vi "AM Modulation Demo (Baseband-Sine) - Template.vi"() -> ()   [LabVIEW 2013]
uses:
  <vilib>/express/express analysis/Spectral/Block/exnSpectralBlock spectral measurements power poly.vi
  <vilib>/express/express analysis/Spectral/Block/exnSpectralBlock spectral measurements power DDT.vi
  <vilib>/express/express analysis/Spectral/XNode/ExpressSpectralMeasurementsBlockNode.xnode
panel:
  in  "WAV Sample Rate":dbl=44100.0 caption="dt"
  in  "Mod. Freq.":dbl=2000.0 caption="Frequency"
  in  "LPF Cut-Off":dbl=10000.0 caption="Lower Cut-Off"
  in  "AWGN (dB)":dbl(slide)=0.6 caption="Standard deviation" scale=-20.0..30.0
  out "Comparision":dynamicdata(graph)
  out "Baseband":dynamicdata(graph)
  out "AM FFT":dynamicdata(graph)
  out "AM Wave":dynamicdata(graph)
  in  "DC Offset":dbl=1.0
  in  "Carrier Amp.":dbl=1.0 caption="Amplitude"
  in  "stop":bool
  in  "Modulation Index":dbl(slide)=1.0 scale=0.0..5.0
  in  "Carrier Freq.":dbl=100000.0 caption="Frequency"
  out "After Rectifier":dynamicdata(graph)=[{"t0"=timestamp(0 s since 1904-01-01), "dt"=10.0, "Y"=array[50000 elements], "attributes"=variant("NI_ChannelName"=variant(string "Sine (Power Spectrum)"), "NI_ExpIsRelativeTime"=variant(bool TRUE), "NI_ExpStartTimeStamp"=variant(timestamp timestamp(3635665779.2842293 s since 1904-01-01)), "NI_ExpTimeStamp"=variant(timestamp timestamp(3635665779.2842293 s since 1904-01-01)), "NI_ExpXDimension"=variant(string "f"), "NI_OriginalChannelName"=variant(string "Sine"))}]
  # "Amplitude Modulation"
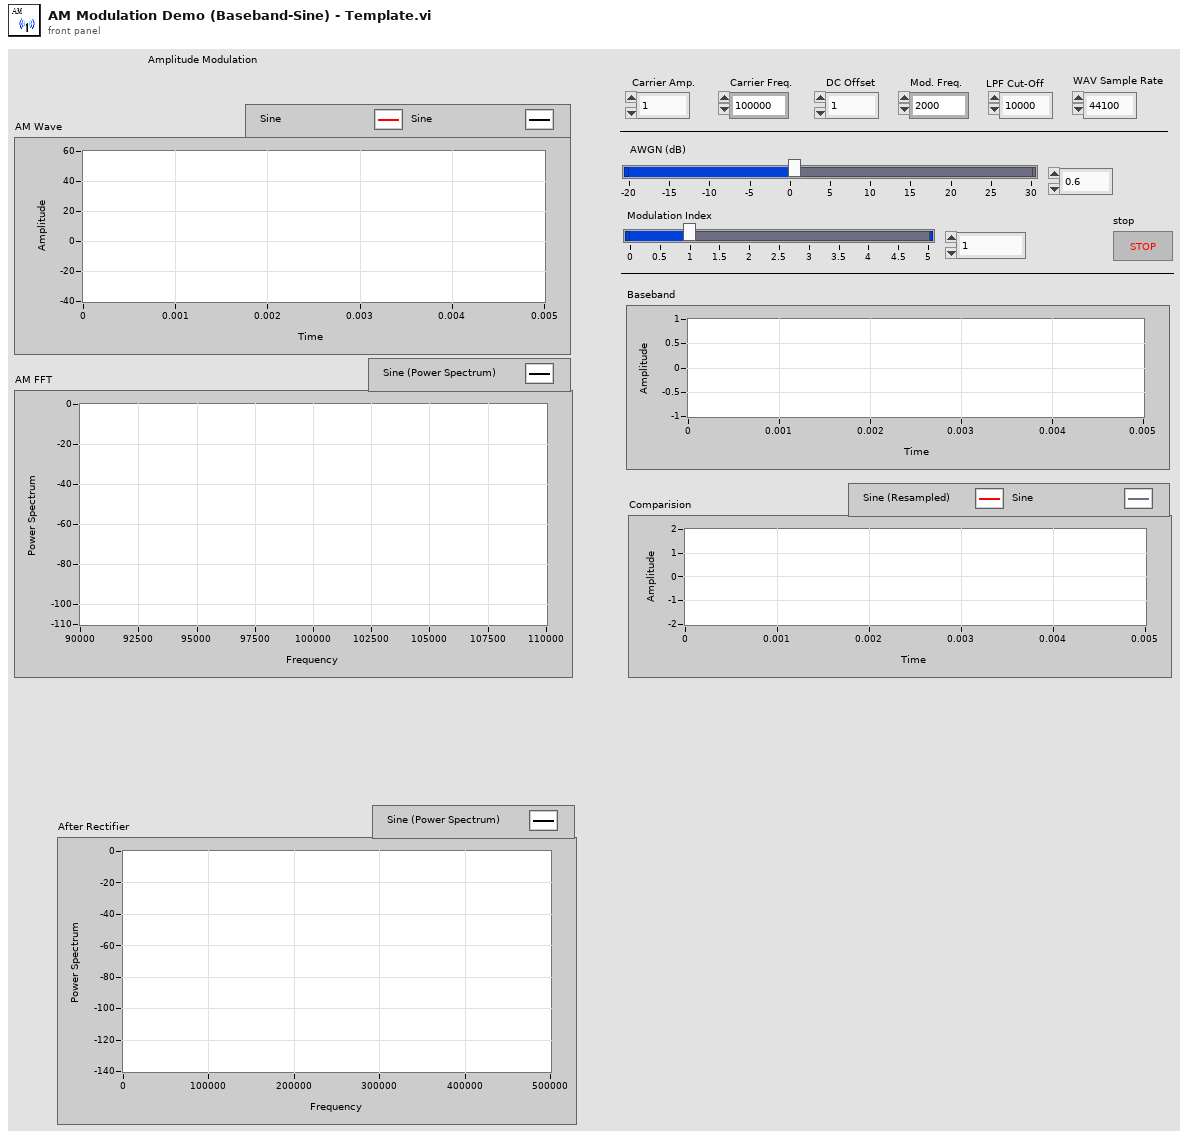
[diagram p1: front panel]
types:
  T1 = cluster{"averaging mode":u16, "weighting mode":u16, "number of averages":u32}
  T2 = cluster{"dB On (F)":bool, "unwrap phase (F)":bool, "convert to degree (F)":bool}
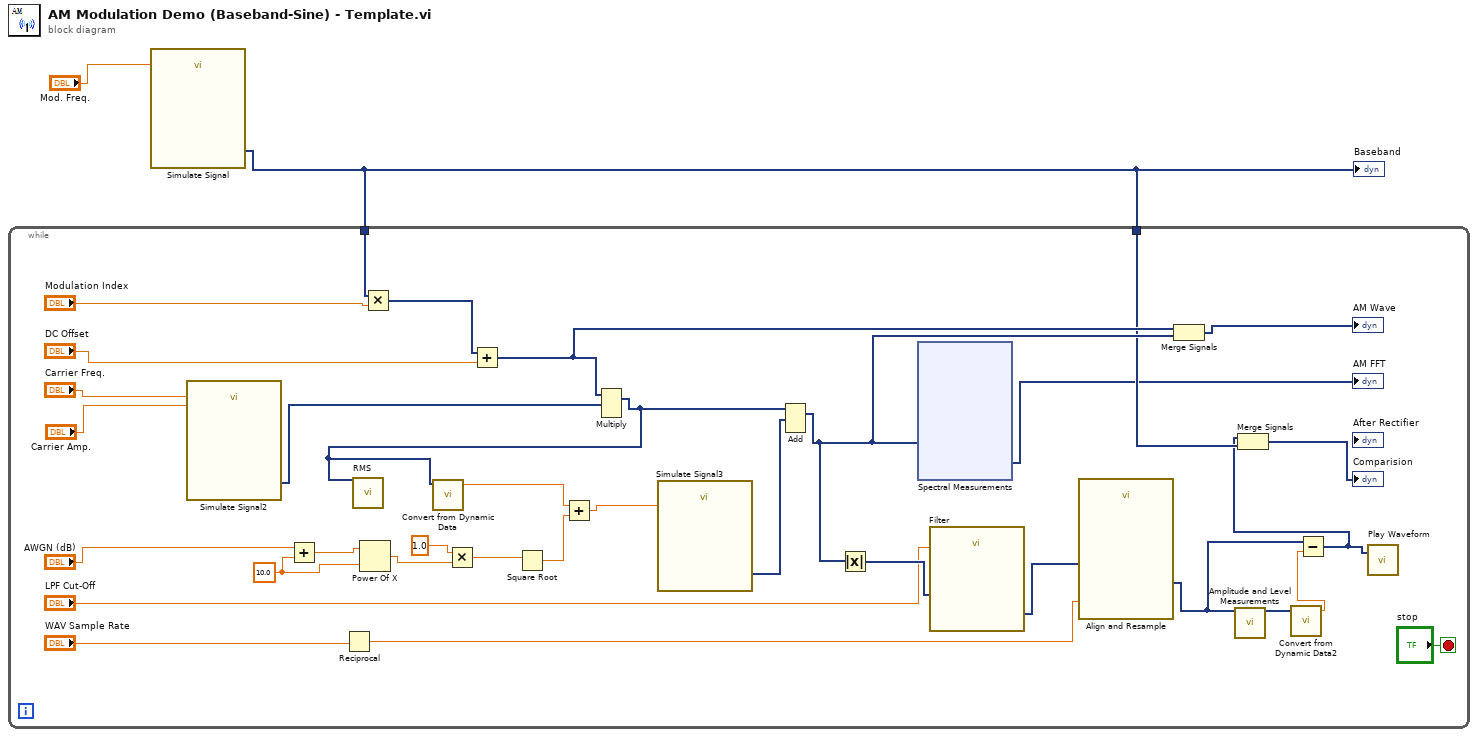
[diagram p0: block diagram]
diagram:
  n1 = call "Simulate Signal"("Frequency"="Mod. Freq.") -> ("Sine"=w1:dynamicdata)  [unwired: 13 in, 1 out]
  "Baseband" <- w1
  n2 = while {
    tunnel: w1 -> [w32]
    tunnel: w1 -> [w5]
    stop <- "stop" stop-if-true
    w26 = 10.0
    n3 = call "Simulate Signal2"("Frequency"="Carrier Freq.", "Amplitude"="Carrier Amp.") -> ("Sine"=w29:dynamicdata)  [unwired: 12 in, 1 out]
    n4 = Add(x="AWGN (dB)", y=w26) -> (x+y=w27:dbl)
    n5 = Reciprocal(x="WAV Sample Rate") -> (1/x=w13:dbl)
    n6 = Power Of X(1:w26, 2:w27) -> (0:w25:dbl)
    n7 = Multiply(x=w32, y="Modulation Index") -> (x*y=w34:dynamicdata)
    n8 = Multiply(x=1.0, y=w25) -> (x*y=w23:dbl)
    n9 = Add(x=w34, y="DC Offset") -> (x+y=w12:dynamicdata)
    n10 = Square Root(x=w23) -> (sqrt(x)=w22:dbl)
    n11 = Multiply(1:w29, 2:w12) -> (0:w18:dynamicdata)  [unwired: 1 in, 1 out]
    n12 = call "RMS"("Signals"=w18) -> ()  [unwired: 13 in, 2 out]
    n13 = call "Convert from Dynamic Data"("Dynamic Data Type"=w18) -> ("Scalar"=w19:dbl)  [unwired: 3 in]
    n14 = Add(x=w19, y=w22) -> (x+y=w21:dbl)
    n15 = call "Simulate Signal3"("Standard deviation"=w21) -> ("DC with Gaussian Noise"=w20:dynamicdata)  [unwired: 13 in, 1 out]
    n16 = Add(1:w20, 2:w18) -> (0:w11:dynamicdata)  [unwired: 1 in, 1 out]
    n17 = Absolute Value(x=w11) -> (abs(x)=w17:dynamicdata)
    n18 = xnode "Spectral Measurements"("Signals"=w11) -> ("Power Spectrum"=→"AM FFT":dynamicdata)  [unwired: 1 in, 1 out]
    n19 = call "Filter"("Lower Cut-Off"="LPF Cut-Off", "Signal"=w17) -> ("Filtered Signal"=w15:dynamicdata)  [unwired: 8 in, 1 out]
    n20 = call "Align and Resample"("dt"=w13, "Signals"=w15) -> ("Resampled Signals"=w7:dynamicdata)  [unwired: 7 in, 2 out]
    n21 = Merge Signals(w12, w11) -> (→"AM Wave":dynamicdata)
    n22 = call "Amplitude and Level Measurements"("Signals"=w7) -> ("Mean (DC)"=w9:dynamicdata)  [unwired: 13 in, 1 out]
    n23 = call "Convert from Dynamic Data2"("Dynamic Data Type"=w9) -> ("Scalar"=w8:dbl)  [unwired: 3 in]
    n24 = Subtract(x=w7, y=w8) -> (x-y=w4:dynamicdata)
    n25 = Merge Signals(w4, w5) -> (→"Comparision":dynamicdata)
    n26 = call "Play Waveform"("Data"=w4) -> ()  [unwired: 18 in, 1 out]
  }
